vi "Timer Vi.vi"(11 "interval (s)":i32=3600) -> (2 "Output":i32, 3 "Samples Collected":i32)   [LabVIEW 2015]
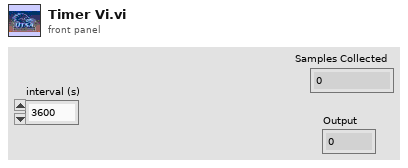
[diagram p1: front panel]
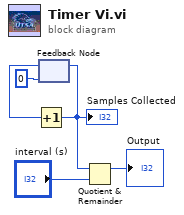
[diagram p0: block diagram]
diagram:
  n1 = feedback #1(0) -> (w1:i32)
  n2 = Increment(x=w1) -> (x+1=w3:i32)
  "Samples Collected" <- w3
  n3 = feedback-in #1(w3) -> ()
  n4 = Quotient & Remainder(x=w3, y="interval (s)") -> (x-y*floor(x/y)=→"Output":i32)  [unwired: 1 out]
